vi "dfd_Set Filter Coef Components.vi"(7 "type":T2, 8 "error in (no error)":errorcluster, 9 "gain":dbl, 10 "coef a (k)":dbl[](array[numeric]), 11 "coef b (v)":dbl[](array[numeric])) -> (0 "error out":errorcluster, 3 "filter coef":T1)   [LabVIEW 2017, in "NI_DigFilterLicensed.lvlib"]
uses:
  <vilib>/addons/Digital Filter Design/NI_DigFilterLicensed.lvlib
  <vilib>/addons/Digital Filter Design/_Objects.llb/DFD Filter Structure Type Selector.ctl
  <vilib>/addons/Digital Filter Design/_Objects.llb/DFD Filter Coef.ctl
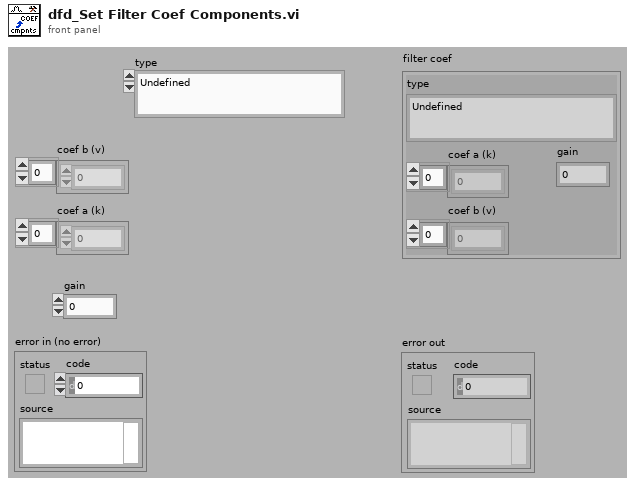
[diagram p1: front panel]
types:
  T1 = typedef "NI_DigFilterLicensed.lvlib/DFD Filter Coef.ctl" = cluster{"type":T2, "gain":dbl, "coef a (k)":dbl[], "coef b (v)":dbl[]}
  T2 = typedef "NI_DigFilterLicensed.lvlib/DFD Filter Structure Type Selector.ctl" = enum16{"Undefined", "FIR Direct Form", "FIR Direct Form Transposed", "FIR Symmetric", "FIR Antisymmetric", "IIR Direct Form I", "IIR Direct Form I Transposed", "IIR Direct Form II", "IIR Direct Form II Transposed", "IIR Cascaded Second Order Sections Form I", "IIR Cascaded Second Order Sections Form I Transposed", "IIR Cascaded Second Order Sections Form II", "IIR Cascaded Second Order Sections Form II Transposed", "Lattice Allpass (basic sections)", "Lattice Allpass (one multiplier sections)", "Lattice Allpass (normalized sections)", "Lattice AR (basic sections)", "Lattice AR (one multiplier sections)", "Lattice AR (normalized sections)", "Lattice MA (minimum phase)", "Lattice MA (maximum phase)", "Lattice ARMA (basic sections)", "Lattice ARMA (one multiplier sections)", "Lattice ARMA (normalized sections)"}
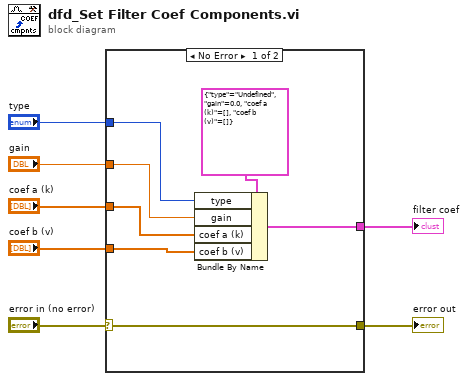
[diagram p0: block diagram]
diagram:
  n1 = case shown="No Error" "error in (no error)" {
    selector: "error in (no error)" -> [w14 w15]
    tunnel: [w14 w15] -> w6
    tunnel: "coef b (v)" -> [w11 _]
    tunnel: "coef a (k)" -> [w10 _]
    tunnel: "gain" -> [w9 _]
    tunnel: "type" -> [w8 _]
    tunnel: [w13 _] -> w1
    frame No Error {
      n2 = Bundle By Name(cluster=T1 {"type"=enum."Undefined", "gain"=0.0, "coef a (k)"=[], "coef b (v)"=[]} ("filter coef"), "type"=w8, "gain"=w9, "coef a (k)"=w10, "coef b (v)"=w11) -> (w13:T1)
    }
    frame Error {
    }
  }
  "error out" <- w6
  "filter coef" <- w1
